vi "Configuration-PromptForChannelParameters_timer.vi"(0 "Control/Feedback\n(Default: False = Feedback)":bool) -> (4 "Poll Time (Out)":u32 caption="Poll Time (ms)" max=600000 step=100, 6 "Parameter (Out)":u8 caption="Poll Type")   [LabVIEW 2015]
panel:
  in  "Poll Type":u8(ring) caption="Parameter" items=["Pulse", "State Low", "State High"]
  in  "OK":bool caption="Quit"
  in  "Poll Time":u32 caption="Poll Time (ms)" max=600000 step=100
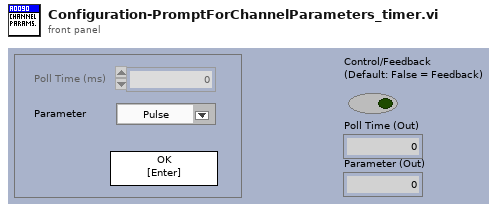
[diagram p1: front panel]
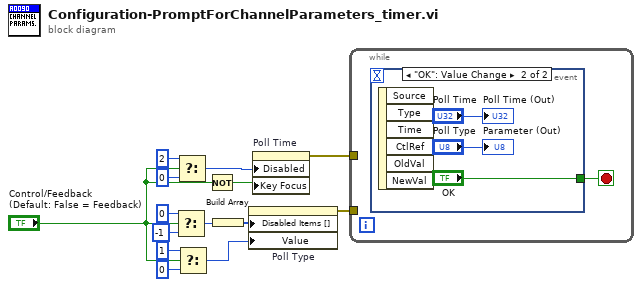
[diagram p0: block diagram]
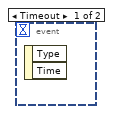
[diagram p2: hidden frame]
diagram:
  n1 = Select(t=0, s="Control/Feedback\n(Default: False = Feedback)", f=-1) -> (s? t:f=w11:i32)
  n2 = Select(t=u8 2, s="Control/Feedback\n(Default: False = Feedback)", f=u8 0) -> (s? t:f=w8:u8)
  n3 = Select(t=u8 1, s="Control/Feedback\n(Default: False = Feedback)", f=u8 0) -> (s? t:f=w2:u8)
  n4 = Not(x="Control/Feedback\n(Default: False = Feedback)") -> (.not. x?=w7:bool)
  n5 = Build Array(w11) -> (w10:i32[])
  n6 = property on="Poll Type" class="Ring (strict)"("Disabled Items []"=w10, "Value"=w2) -> (error out=w9:errorcluster)  [unwired: 2 in, 1 out]
  n7 = property on="Poll Time" class="DigNum (strict)"("Disabled"=w8, "Key Focus"=w7) -> (error out=w14:errorcluster)  [unwired: 2 in, 1 out]
  n8 = while {
    tunnel: w14 -> [_]
    tunnel: w9 -> [_]
    stop <- w15 stop-if-true
    n9 = event shown="[1] \"OK\": Value Change" {
      selector: _ -> [_ _]
      dyn-events: _ -> [_ _]
      timeout: _ -> [_ _]
      tunnel: [_ "OK"] -> w15
      event Timeout {
        n10 = event-data() -> ()  [unwired: 1 in, 2 out]
      }
      event "OK": Value Change {
        n11 = event-data() -> ()  [unwired: 1 in, 6 out]
        "Poll Time (Out)" <- "Poll Time"
        "Parameter (Out)" <- "Poll Type"
      }
    }
  }
